vi "CoboltLaser_ComPortClose.vi"(0 "ComPort":refnum<visa-resource-name>, 5 "error in (no error)":errorcluster) -> (19 "error out":errorcluster)   [LabVIEW 2019]
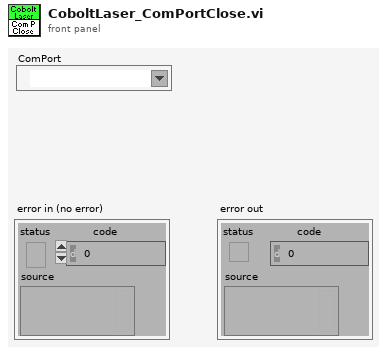
[diagram p1: front panel]
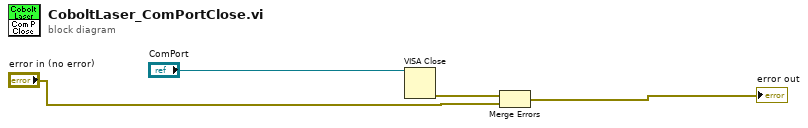
[diagram p0: block diagram]
diagram:
  n1 = VISA Close(VISA resource name="ComPort") -> (error out=w4:errorcluster)  [unwired: 1 in]
  n2 = Merge Errors(w4, "error in (no error)") -> (→"error out":errorcluster)
